vi "RxTx.vi"(8 "error in (no error)":errorcluster) -> (0 "error out":errorcluster)   [LabVIEW 2018]
uses:
  RxTx/RxTx.lvclass
  RxTx/RxTx.lvclass/RxTx.ctl
  <vilib>/addons/_JKI Toolkits/Caraya/classes/Assert/Assert Equal Value_Variant.vi
  <vilib>/addons/_JKI Toolkits/Caraya/classes/Assert/Assert Error.vi
  <vilib>/addons/_JKI Toolkits/Caraya/classes/Test/Test.lvclass
  <vilib>/addons/_JKI Toolkits/Caraya/classes/Assert/Assert.lvclass
panel:
  in  "RxTx in":refnum<class "RxTx.lvclass">
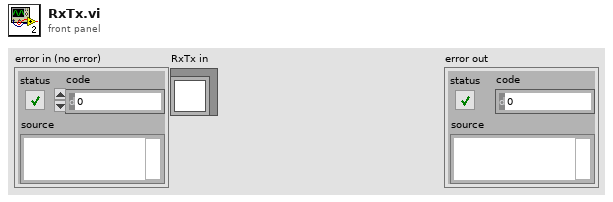
[diagram p1: front panel]
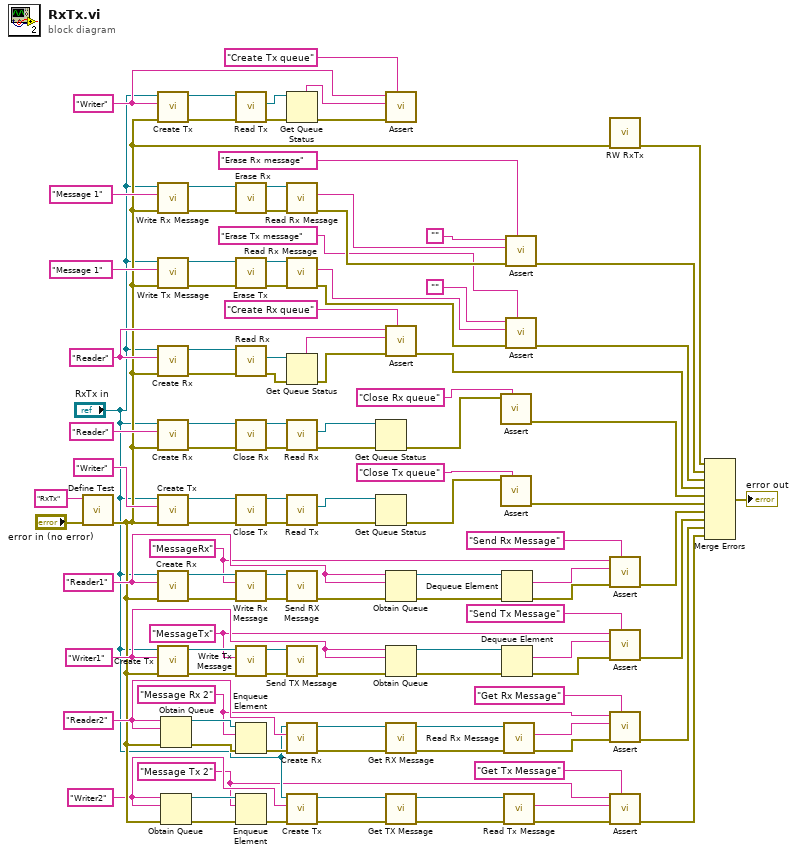
[diagram p0: block diagram]
diagram:
  w2 = "Message Tx 2" ("Rx Message")
  w10 = "Writer2" ("Rx Message")
  w18 = "Message Rx 2" ("Rx Message")
  w25 = "Reader2" ("Rx Message")
  w31 = "MessageTx" ("Rx Message")
  w33 = "Writer1" ("Rx Message")
  w45 = "MessageRx" ("Rx Message")
  w49 = "Reader1" ("Rx Message")
  w82 = "Writer" ("Rx Message")
  w85 = "Reader" ("Rx Message")
  n1 = call <vilib>:"Define Test.vi"("error in (no error)"="error in (no error)", "Label (VI Title)"="RxTx") -> ("error out"=w13:errorcluster)  [unwired: 8 in, 1 out]
  n2 = call "Create Tx.vi"("error in (no error)"=w13, "Writer Name"=w82, "RxTx in"="RxTx in") -> ("error out"=w76:errorcluster, "RxTx out"=w77:refnum<class "RxTx.lvclass">)  [unwired: 7 in]
  n3 = call "Write Rx Message.vi"("error in (no error)"=w13, "Rx Message"="Message 1", "RxTx in"="RxTx in") -> ("error out"=w111:errorcluster, "RxTx out"=w110:refnum<class "RxTx.lvclass">)  [unwired: 7 in]
  n4 = call "Write Tx Message.vi"("error in (no error)"=w13, "Tx Message"="Message 1" ("Rx Message"), "RxTx in"="RxTx in") -> ("error out"=w97:errorcluster, "RxTx out"=w96:refnum<class "RxTx.lvclass">)  [unwired: 7 in]
  n5 = call "Create Rx.vi"("error in (no error)"=w13, "Reader Name"=w85, "RxTx in"="RxTx in") -> ("error out"=w91:errorcluster, "RxTx out"=w90:refnum<class "RxTx.lvclass">)  [unwired: 7 in]
  n6 = call "Create Rx.vi"("error in (no error)"=w13, "Reader Name"="Reader" ("Rx Message"), "RxTx in"="RxTx in") -> ("error out"=w73:errorcluster, "RxTx out"=w72:refnum<class "RxTx.lvclass">)  [unwired: 7 in]
  n7 = call "Create Tx.vi"("error in (no error)"=w13, "Writer Name"="Writer" ("Rx Message"), "RxTx in"="RxTx in") -> ("error out"=w64:errorcluster, "RxTx out"=w63:refnum<class "RxTx.lvclass">)  [unwired: 7 in]
  n8 = call "Create Rx.vi"("error in (no error)"=w13, "Reader Name"=w49, "RxTx in"="RxTx in") -> ("error out"=w54:errorcluster, "RxTx out"=w51:refnum<class "RxTx.lvclass">)  [unwired: 7 in]
  n9 = call "Create Tx.vi"("error in (no error)"=w13, "Writer Name"=w33, "RxTx in"="RxTx in") -> ("error out"=w41:errorcluster, "RxTx out"=w40:refnum<class "RxTx.lvclass">)  [unwired: 7 in]
  n10 = Obtain Queue(name (unnamed)=w25, element data type=w25, error in (no error)=w13) -> (queue out=w27:refnum<queue>, error out=w28:errorcluster)  [unwired: 2 in, 1 out]
  n11 = Obtain Queue(name (unnamed)=w10, element data type=w10, error in (no error)=w13) -> (queue out=w15:refnum<queue>, error out=w14:errorcluster)  [unwired: 2 in, 1 out]
  n12 = call "Read Tx.vi"("error in (no error)"=w76, "RxTx in"=w77) -> ("error out"=w79:errorcluster, "Tx"=w78:refnum<queue>)  [unwired: 7 in, 1 out]
  n13 = call "Erase Rx.vi"("error in (no error)"=w111, "RxTx in"=w110) -> ("error out"=w109:errorcluster, "RxTx out"=w104:refnum<class "RxTx.lvclass">)  [unwired: 8 in]
  n14 = call "Erase Tx.vi"("error in (no error)"=w97, "RxTx in"=w96) -> ("error out"=w94:errorcluster, "RxTx out"=w95:refnum<class "RxTx.lvclass">)  [unwired: 8 in]
  n15 = call "Read Rx.vi"("error in (no error)"=w91, "RxTx in"=w90) -> ("error out"=w88:errorcluster, "Rx"=w89:refnum<queue>)  [unwired: 7 in, 1 out]
  n16 = call "Close Rx.vi"("error in (no error)"=w73, "RxTx in"=w72) -> ("error out"=w71:errorcluster, "RxTx out"=w70:refnum<class "RxTx.lvclass">)  [unwired: 8 in]
  n17 = call "Close Tx.vi"("error in (no error)"=w64, "RxTx in"=w63) -> ("error out"=w61:errorcluster, "RxTx out"=w60:refnum<class "RxTx.lvclass">)  [unwired: 8 in]
  n18 = call "Write Rx Message.vi"("error in (no error)"=w54, "Rx Message"=w45, "RxTx in"=w51) -> ("error out"=w53:errorcluster, "RxTx out"=w52:refnum<class "RxTx.lvclass">)  [unwired: 7 in]
  n19 = call "Write Tx Message.vi"("error in (no error)"=w41, "Tx Message"=w31, "RxTx in"=w40) -> ("error out"=w39:errorcluster, "RxTx out"=w38:refnum<class "RxTx.lvclass">)  [unwired: 7 in]
  n20 = Enqueue Element(queue=w27, element=w18, error in (no error)=w28) -> (error out=w26:errorcluster)  [unwired: 1 in, 2 out]
  n21 = Enqueue Element(queue=w15, element=w2, error in (no error)=w14) -> (error out=w12:errorcluster)  [unwired: 1 in, 2 out]
  n22 = Get Queue Status(queue=w78, error in (no error)=w79) -> (queue name=w81:string, error out=w80:errorcluster)  [unwired: 1 in, 6 out]
  n23 = call "Read Rx Message.vi"("error in (no error)"=w109, "RxTx in"=w104) -> ("error out"=w108:errorcluster, "Rx Message"=w107:string)  [unwired: 7 in, 1 out]
  n24 = call "Read Rx Message.vi"("error in (no error)"=w94, "RxTx in"=w95) -> ("error out"=w98:errorcluster, "Rx Message"=w99:string)  [unwired: 7 in, 1 out]
  n25 = Get Queue Status(queue=w89, error in (no error)=w88) -> (queue name=w86:string, error out=w87:errorcluster)  [unwired: 1 in, 6 out]
  n26 = call "Read Rx.vi"("error in (no error)"=w71, "RxTx in"=w70) -> ("error out"=w67:errorcluster, "Rx"=w69:refnum<queue>)  [unwired: 7 in, 1 out]
  n27 = call "Read Tx.vi"("error in (no error)"=w61, "RxTx in"=w60) -> ("error out"=w58:errorcluster, "Tx"=w59:refnum<queue>)  [unwired: 7 in, 1 out]
  n28 = call "Send RX Message.vi"("error in (no error)"=w53, "RxTx in"=w52) -> ("error out"=w50:errorcluster)  [unwired: 8 in, 1 out]
  n29 = call "Send TX Message.vi"("error in (no error)"=w39, "RxTx in"=w38) -> ("error out"=w37:errorcluster)  [unwired: 8 in, 1 out]
  n30 = call "Create Rx.vi"("error in (no error)"=w26, "Reader Name"=w25, "RxTx in"="RxTx in") -> ("error out"=w24:errorcluster, "RxTx out"=w23:refnum<class "RxTx.lvclass">)  [unwired: 7 in]
  n31 = call "Create Tx.vi"("error in (no error)"=w12, "Writer Name"=w10, "RxTx in"="RxTx in") -> ("error out"=w8:errorcluster, "RxTx out"=w9:refnum<class "RxTx.lvclass">)  [unwired: 7 in]
  n32 = Get Queue Status(queue=w69, error in (no error)=w67) -> (error out=w68:errorcluster)  [unwired: 1 in, 7 out]
  n33 = Get Queue Status(queue=w59, error in (no error)=w58) -> (error out=w57:errorcluster)  [unwired: 1 in, 7 out]
  n34 = call-poly <vilib>:"Assert.vi"("Label"="Create Tx queue" ("Label (VI Title)"), "error in (no error)"=w80, "Actual"=w81, "Expected"=w82) -> ()  [unwired: 6 in, 2 out]
  n35 = call-poly <vilib>:"Assert.vi"("Label"="Create Rx queue" ("Label (VI Title)"), "error in (no error)"=w87, "Actual"=w86, "Expected"=w85) -> ("error out"=w84:errorcluster)  [unwired: 6 in, 1 out]
  n36 = Obtain Queue(name (unnamed)=w49, element data type=w49, error in (no error)=w50) -> (queue out=w48:refnum<queue>, error out=w47:errorcluster)  [unwired: 2 in, 1 out]
  n37 = Obtain Queue(name (unnamed)=w33, element data type=w33, error in (no error)=w37) -> (queue out=w34:refnum<queue>, error out=w36:errorcluster)  [unwired: 2 in, 1 out]
  n38 = call "Get RX Message.vi"("error in (no error)"=w24, "RxTx in"=w23) -> ("error out"=w22:errorcluster, "RxTx out"=w21:refnum<class "RxTx.lvclass">)  [unwired: 8 in]
  n39 = call "Get TX Message.vi"("error in (no error)"=w8, "RxTx in"=w9) -> ("error out"=w7:errorcluster, "RxTx out"=w6:refnum<class "RxTx.lvclass">)  [unwired: 8 in]
  n40 = call-poly <vilib>:"Assert.vi"("Label"="Close Rx queue" ("Label (VI Title)"), "Error?"=w68) -> ("error out"=w66:errorcluster)  [unwired: 8 in, 1 out]
  n41 = call-poly <vilib>:"Assert.vi"("Label"="Close Tx queue" ("Label (VI Title)"), "Error?"=w57) -> ("error out"=w56:errorcluster)  [unwired: 8 in, 1 out]
  n42 = Dequeue Element(queue=w48, error in (no error)=w47) -> (element=w46:string, error out=w44:errorcluster)  [unwired: 1 in, 2 out]
  n43 = Dequeue Element(queue=w34, error in (no error)=w36) -> (element=w32:string, error out=w35:errorcluster)  [unwired: 1 in, 2 out]
  n44 = call "Read Rx Message.vi"("error in (no error)"=w22, "RxTx in"=w21) -> ("error out"=w20:errorcluster, "Rx Message"=w19:string)  [unwired: 7 in, 1 out]
  n45 = call "Read Tx Message.vi"("error in (no error)"=w7, "RxTx in"=w6) -> ("error out"=w5:errorcluster, "Tx Message"=w3:string)  [unwired: 7 in, 1 out]
  n46 = call-poly <vilib>:"Assert.vi"("Label"="Erase Rx message" ("Label (VI Title)"), "error in (no error)"=w108, "Actual"=w107, "Expected"="") -> ("error out"=w103:errorcluster)  [unwired: 6 in, 1 out]
  n47 = call-poly <vilib>:"Assert.vi"("Label"="Erase Tx message" ("Label (VI Title)"), "error in (no error)"=w98, "Actual"=w99, "Expected"="") -> ("error out"=w93:errorcluster)  [unwired: 6 in, 1 out]
  n48 = call "RW RxTx.vi"("error in (no error)"=w13) -> ("error out"=w113:errorcluster)  [unwired: 10 in]
  n49 = call-poly <vilib>:"Assert.vi"("Label"="Send Rx Message" ("Label (VI Title)"), "error in (no error)"=w44, "Actual"=w46, "Expected"=w45) -> ("error out"=w43:errorcluster)  [unwired: 6 in, 1 out]
  n50 = call-poly <vilib>:"Assert.vi"("Label"="Send Tx Message" ("Label (VI Title)"), "error in (no error)"=w35, "Actual"=w32, "Expected"=w31) -> ("error out"=w29:errorcluster)  [unwired: 6 in, 1 out]
  n51 = call-poly <vilib>:"Assert.vi"("Label"="Get Rx Message" ("Label (VI Title)"), "error in (no error)"=w20, "Actual"=w19, "Expected"=w18) -> ("error out"=w17:errorcluster)  [unwired: 6 in, 1 out]
  n52 = call-poly <vilib>:"Assert.vi"("Label"="Get Tx Message" ("Label (VI Title)"), "error in (no error)"=w5, "Actual"=w3, "Expected"=w2) -> ("error out"=w4:errorcluster)  [unwired: 6 in, 1 out]
  n53 = Merge Errors(w113, w103, w93, w84, w66, w56, w43, w29, w17, w4) -> (→"error out":errorcluster)
